vi "UMLEditor export_Windows.vi"(1 "PrinterName":string, 2 "path":path, 3 "PaperSize":i32, 4 "orientation":u16, 5 "error in":errorcluster, 6 "copies":i32) -> (19 "error out":errorcluster)   [LabVIEW 2010]
panel:
  in  "NIReports.Report":refnum<k7>
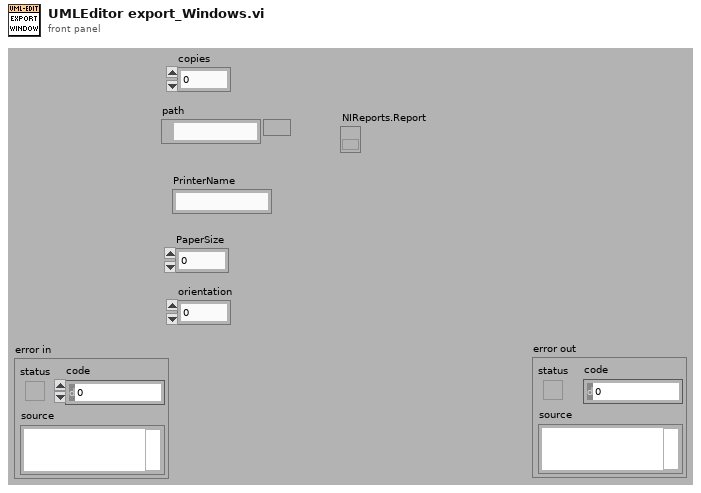
[diagram p1: front panel]
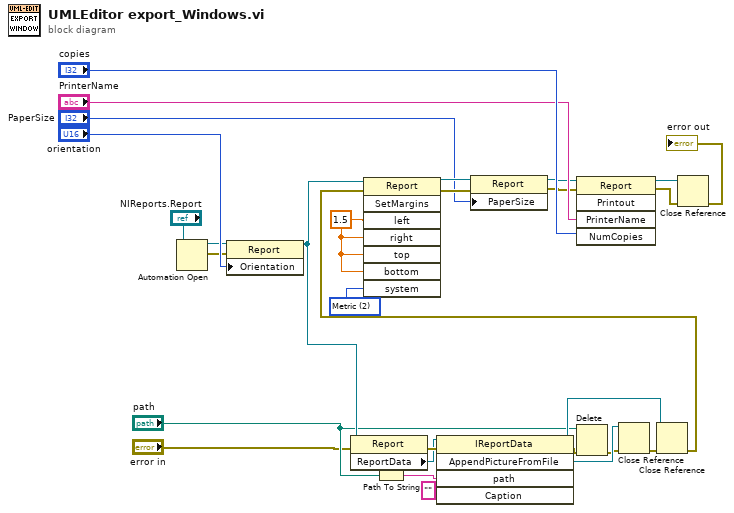
[diagram p0: block diagram]
diagram:
  w27 = 1.5 ("left")
  w26 = 2 items=["Default", "US", "Metric"] ("system")
  n1 = Automation Open(Automation Refnum="NIReports.Report") -> (Automation Refnum=w2:refnum<k7>, error out=w13:errorcluster)  [unwired: 1 in, 2 out]
  n2 = property class="Report"(reference=w2, error in=w13, "Orientation"="orientation") -> (reference out=w24:refnum<k7>)  [unwired: 1 out]
  n3 = property class="Report"(reference=w24, error in="error in") -> (error out=w5:errorcluster, "ReportData"=w3:refnum<k7>)  [unwired: 1 out]
  n4 = Path To String(path="path") -> (string=w6:string)
  n5 = invoke class="IReportData" method="AppendPictureFromFile"(reference=w3, error in=w5, "path"=w6, "Caption"="") -> (reference out=w12:refnum<k7>, error out=w8:errorcluster, "AppendPictureFromFile"=w11:refnum<k7>)  [unwired: 1 in, 2 out]
  n6 = Delete(path (use dialog)="path", error in=w8) -> (error out=w10:errorcluster)  [unwired: 5 out]
  n7 = Close Reference(reference=w11, error in (no error)=w10) -> (error out=w9:errorcluster)
  n8 = Close Reference(reference=w12, error in (no error)=w9) -> (error out=w25:errorcluster)
  n9 = invoke class="Report" method="SetMargins"(reference=w24, error in=w25, "left"=w27, "right"=w27, "top"=w27, "bottom"=w27, "system"=w26) -> (reference out=w22:refnum<k7>, error out=w23:errorcluster)  [unwired: 1 in, 6 out]
  n10 = property class="Report"(reference=w22, error in=w23, "PaperSize"="PaperSize") -> (reference out=w18:refnum<k7>, error out=w19:errorcluster)
  n11 = invoke class="Report" method="Printout"(reference=w18, error in=w19, "PrinterName"="PrinterName", "NumCopies"="copies") -> (reference out=w14:refnum<k7>, error out=w15:errorcluster)  [unwired: 1 in, 3 out]
  n12 = Close Reference(reference=w14, error in (no error)=w15) -> (error out=→"error out":errorcluster)
